vi "Disable-Enable scrollbars.vi"(8 "error in (no error)":errorcluster, 11 "Disabled state":T1(ring)=enum."Disabled and Grayed Out") -> (0 "error out":errorcluster)   [LabVIEW 2013]
uses:
  Globals/gl_Time series viewer globals.vi
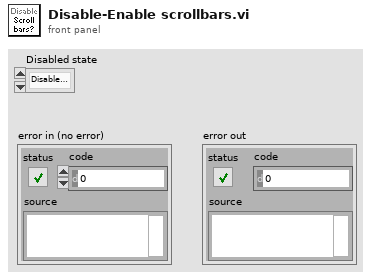
[diagram p1: front panel]
types:
  T1 = enum8{"Enabled", "Disabled", "Disabled and Grayed Out"}
  T2 = typedef "Timelapse viewer refs.ctl" = cluster{"This VI":refnum<vi>, "AVI Mode ind":refnum<vi>, "Play":refnum<vi>, "Stop":refnum<vi>, "Back":refnum<vi>, "Scrollbar":refnum<vi>, "Video length info":refnum<vi>, "Expected speed values":refnum<vi>, "Intensity":refnum<vi>, "Path":refnum<vi>, "Selection sliders":refnum<vi>, "Speed Graph ref":refnum<vi>, "Frame rate set (fps)":refnum<vi>}
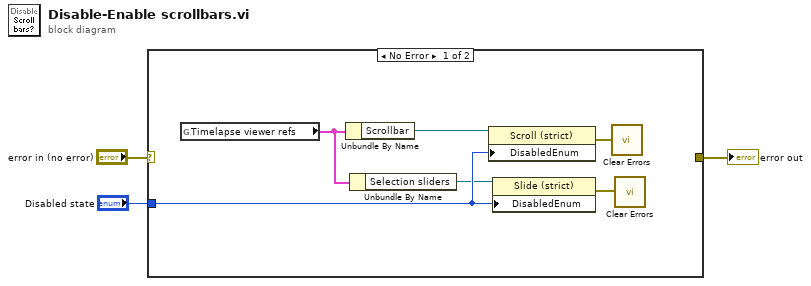
[diagram p0: block diagram]
diagram:
  n1 = case shown="No Error" "error in (no error)" {
    selector: "error in (no error)" -> [_ w10]
    tunnel: "Disabled state" -> [w9 _]
    tunnel: [_ w10] -> w1
    frame No Error {
      n2 = global read "gl_Time series viewer globals.vi" "Timelapse viewer refs"() -> (w7:T2)
      n3 = Unbundle By Name(w7) -> ("Scrollbar"=w6:refnum<vi>)
      n4 = Unbundle By Name(w7) -> ("Selection sliders"=w8:refnum<vi>)
      n5 = property on="Property Node" class="Scroll (strict)"(reference=w6, "DisabledEnum"=w9) -> (error out=w4:errorcluster)  [unwired: 1 in, 1 out]
      n6 = property on="Property Node" class="Slide (strict)"(reference=w8, "DisabledEnum"=w9) -> (error out=w5:errorcluster)  [unwired: 1 in, 1 out]
      n7 = call <vilib>:"Clear Errors.vi"("error in (no error)"=w4) -> ()  [unwired: 6 in, 1 out]
      n8 = call <vilib>:"Clear Errors.vi"("error in (no error)"=w5) -> ()  [unwired: 6 in, 1 out]
    }
    frame Error {
    }
  }
  "error out" <- w1
